vi "Test Wait_For_LACK_OF_activity.vi"() -> ()   [LabVIEW 2013]
panel:
  in  "Stop Button":bool
  out "Rev String":string
  in  "String In":string
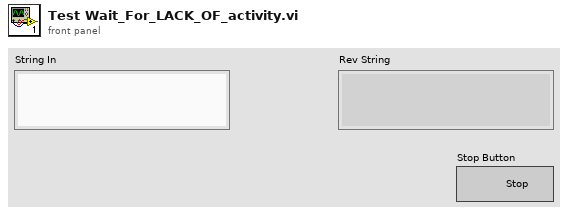
[diagram p1: front panel]
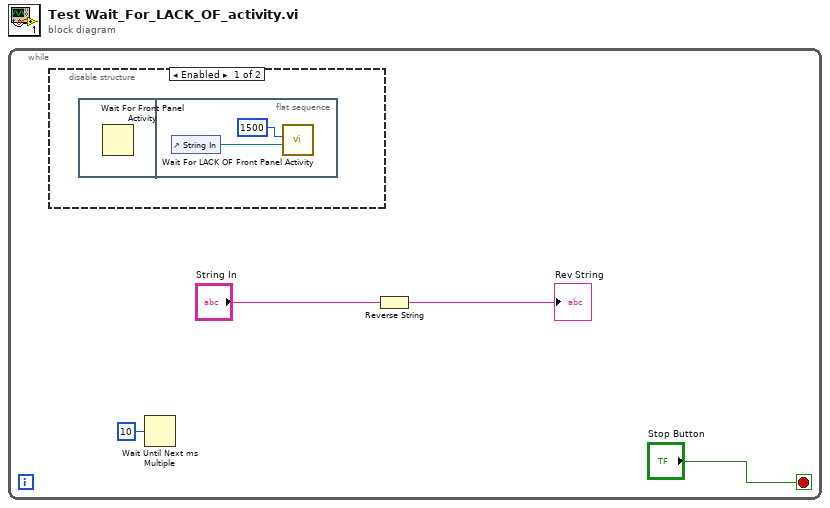
[diagram p0: block diagram]
diagram:
  n1 = while {
    stop <- "Stop Button" stop-if-true
    n2 = disable-structure shown="Enabled" {
      frame Enabled {
        n3 = flat-sequence {
          frame #0 {
            n4 = Wait For Front Panel Activity() -> ()  [unwired: 3 in, 1 out]
          }
          frame #1 {
            n5 = control-ref of="String In"() -> (w5:refnum<vi>)
            n6 = call "Wait For LACK OF Front Panel Activity.vi"("Delay (ms)"=1500, "Generic VI Reference"=w5) -> ()  [unwired: 9 in]
          }
        }
      }
      frame Disabled {
      }
    }
    n7 = Wait Until Next ms Multiple(millisecond multiple=u32 10) -> ()  [unwired: 1 out]
    n8 = Reverse String(1:"String In") -> (0:→"Rev String":string)
  }
